vi "Status_Frame.vi"(8 "error in (no error)":errorcluster, 11 "Motor Control DevRef":T1={"DeviceStatus"={"status"=FALSE, "code"=0, "source"=""}, "Type"=enum."PWM", "PWM"={"PWM Channel"=enum."PWM 1", "DeadBand"={"Name"="", "maxPositivePwm"=0, "minPositivePwm"=0, "centerPwm"=0, "maxNegativePwm"=0, "minNegativePwm"=0, "angularRange"=0}}, "CAN"={"Device Number"=0, "SetOutput VI Ref"=variant(enum8{"Percent VBus", "Current", "Speed", "Position", "Voltage"} enum."Percent VBus"), "GetOutput VI Ref"=variant(refnum<k1> refnum), "Enable VI Ref"=variant(dbl 12.0), "Disable VI Ref"=variant(enum8{"Percent VBus", "Speed", "Position", "Slave", "Unchanged / Invalid", "Voltage Compensation", "Current", "Motion Profile"} enum."Percent VBus"), "Data"=variant}, "Invert"=FALSE, "DIO PWM"={"PWM \"Enable\" Channel"=enum."Invalid", "DIOChannel"=enum."Invalid", "PWM Rate"=0.0}}) -> (0 "error out":errorcluster, 3 "PhoenixMotorControlDevRef":T1={"DeviceStatus"={"status"=FALSE, "code"=0, "source"=""}, "Type"=enum."PWM", "PWM"={"PWM Channel"=enum."PWM 1", "DeadBand"={"Name"="", "maxPositivePwm"=0, "minPositivePwm"=0, "centerPwm"=0, "maxNegativePwm"=0, "minNegativePwm"=0, "angularRange"=0}}, "CAN"={"Device Number"=0, "SetOutput VI Ref"=variant(enum8{"Percent VBus", "Current", "Speed", "Position", "Voltage"} enum."Percent VBus"), "GetOutput VI Ref"=variant(refnum<k1> refnum), "Enable VI Ref"=variant(dbl 12.0), "Disable VI Ref"=variant(enum8{"Percent VBus", "Speed", "Position", "Slave", "Unchanged / Invalid", "Voltage Compensation", "Current", "Motion Profile"} enum."Percent VBus"), "Data"=variant}, "Invert"=FALSE, "DIO PWM"={"PWM \"Enable\" Channel"=enum."Invalid", "DIOChannel"=enum."Invalid", "PWM Rate"=0.0}})   [LabVIEW 2020]
uses:
  <vilib>/Rock Robotics/WPI/MotorControl/WPI_MotorControlDeviceRef.ctl
  <vilib>/Rock Robotics/WPI/MotorControl/WPI_MotorControlType.ctl
  <vilib>/Rock Robotics/SystemInterfaces/DIO/FPGA_DIOPWMChannel.ctl
  <vilib>/Rock Robotics/WPI/PWM/WPI_PWMDeadband.ctl
  <vilib>/Rock Robotics/SystemInterfaces/DIO/FPGA_DIOChannel.ctl
  <vilib>/Rock Robotics/WPI/ThirdParty/Phoenix-LabVIEW/Motor Controller/Controls/CTRE_Phoenix_MotorControl_StatusFrameEnhanced.ctl
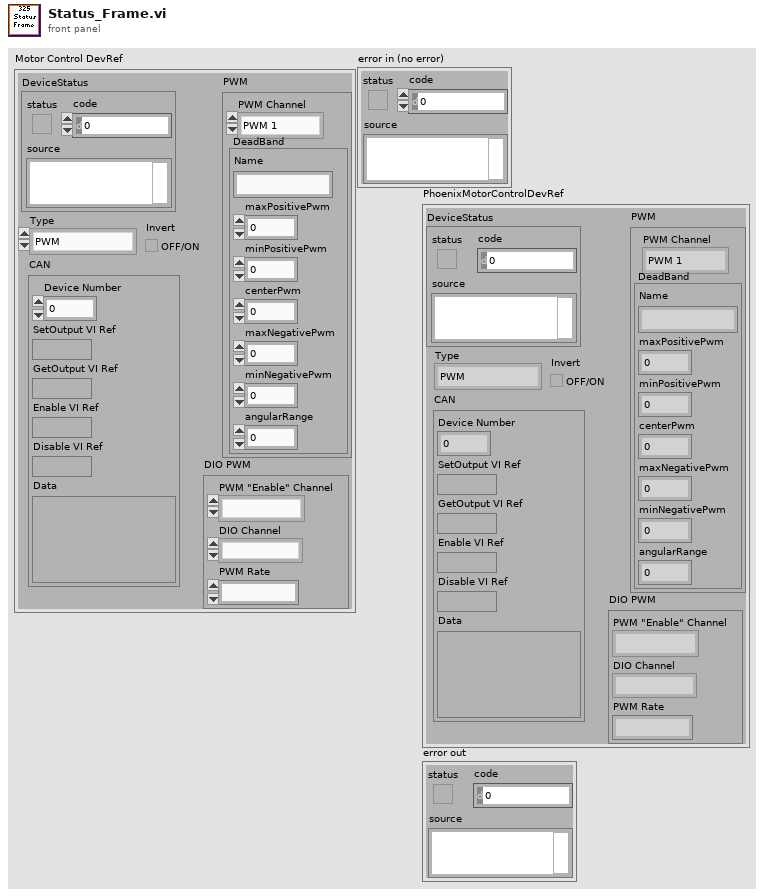
[diagram p1: front panel]
types:
  T1 = typedef "WPI_MotorControlDeviceRef.ctl" = cluster{"DeviceStatus":errorcluster, "Type":T2, "PWM":cluster{"PWM Channel":T3, "DeadBand":T4}, "CAN":cluster{"Device Number":u8, "SetOutput VI Ref":variant, "GetOutput VI Ref":variant, "Enable VI Ref":variant, "Disable VI Ref":variant, "Data":variant}, "Invert":bool, "DIO PWM":cluster{"PWM \"Enable\" Channel":T3, "DIOChannel":T5, "PWM Rate":dbl}}
  T2 = typedef "WPI_MotorControlType.ctl" = enum16{"PWM", "CAN", "DIO PWM"}
  T3 = typedef "FPGA_DIOPWMChannel.ctl" = enum8{"PWM 0", "PWM 1", "PWM 2", "PWM 3", "PWM 4", "PWM 5", "PWM 6", "PWM 7", "PWM 8", "PWM 9", "PWM MXP 0", "PWM MXP 1", "PWM MXP 2", "PWM MXP 3", "PWM MXP 4", "PWM MXP 5", "PWM MXP 6", "PWM MXP 7", "PWM MXP 8", "PWM MXP 9", "Invalid"}
  T4 = typedef "WPI_PWMDeadband.ctl" = cluster{"Name":string, "maxPositivePwm":i32, "minPositivePwm":i32, "centerPwm":i32, "maxNegativePwm":i32, "minNegativePwm":i32, "angularRange":u16}
  T5 = typedef "FPGA_DIOChannel.ctl" = enum8{"DIO 0", "DIO 1", "DIO 2", "DIO 3", "DIO 4", "DIO 5", "DIO 6", "DIO 7", "DIO 8", "DIO 9", "DIO MXP 0", "DIO MXP 1", "DIO MXP 2", "DIO MXP 3", "DIO MXP 4", "DIO MXP 5", "DIO MXP 6", "DIO MXP 7", "DIO MXP 8", "DIO MXP 9", "DIO MXP 10", "DIO MXP 11", "DIO MXP 12", "DIO MXP 13", "DIO MXP 14", "DIO MXP 15", "SPI Port CS1", "SPI Port CS2", "SPI Port CS3", "SPI Port MISO", "SPI Port MOSI", "Invalid"}
  T6 = typedef "CTRE_Phoenix_MotorControl_StatusFrameEnhanced.ctl" = u16
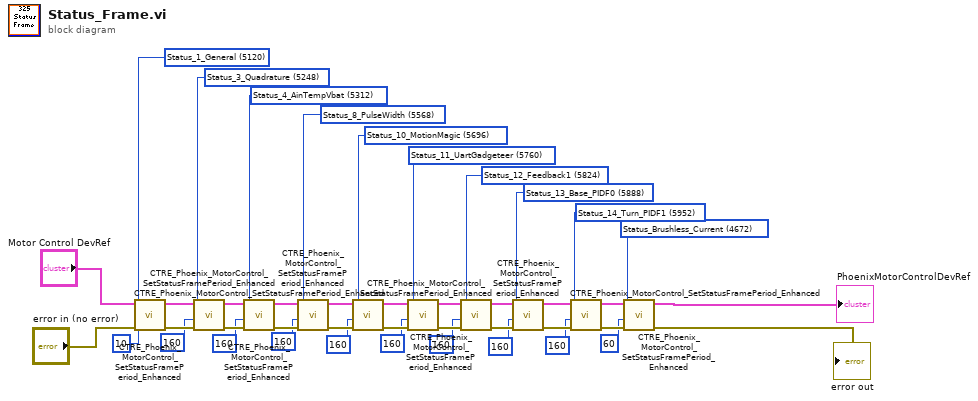
[diagram p0: block diagram]
diagram:
  w11 = T6 4672 items=["Status_1_General"=5120, "Status_2_Feedback0"=5184, "Status_3_Quadrature"=5248, "Status_4_AinTempVbat"=5312, "Status_6_Misc"=5440, "Status_7_CommStatus"=5504, "Status_8_PulseWidth"=5568, "Status_9_MotProfBuffer"=5632, "Status_10_MotionMagic"=5696, "Status_11_UartGadgeteer"=5760, "Status_12_Feedback1"=5824, "Status_13_Base_PIDF0"=5888, "Status_14_Turn_PIDF1"=5952, "Status_15_FirmwareApiStatus"=6016, "Status_Brushless_Current"=4672] ("Status Frame")
  w12 = T6 5952 items=["Status_1_General"=5120, "Status_2_Feedback0"=5184, "Status_3_Quadrature"=5248, "Status_4_AinTempVbat"=5312, "Status_6_Misc"=5440, "Status_7_CommStatus"=5504, "Status_8_PulseWidth"=5568, "Status_9_MotProfBuffer"=5632, "Status_10_MotionMagic"=5696, "Status_11_UartGadgeteer"=5760, "Status_12_Feedback1"=5824, "Status_13_Base_PIDF0"=5888, "Status_14_Turn_PIDF1"=5952, "Status_15_FirmwareApiStatus"=6016, "Status_Brushless_Current"=4672] ("Status Frame")
  w13 = T6 5888 items=["Status_1_General"=5120, "Status_2_Feedback0"=5184, "Status_3_Quadrature"=5248, "Status_4_AinTempVbat"=5312, "Status_6_Misc"=5440, "Status_7_CommStatus"=5504, "Status_8_PulseWidth"=5568, "Status_9_MotProfBuffer"=5632, "Status_10_MotionMagic"=5696, "Status_11_UartGadgeteer"=5760, "Status_12_Feedback1"=5824, "Status_13_Base_PIDF0"=5888, "Status_14_Turn_PIDF1"=5952, "Status_15_FirmwareApiStatus"=6016, "Status_Brushless_Current"=4672] ("Status Frame")
  w14 = T6 5824 items=["Status_1_General"=5120, "Status_2_Feedback0"=5184, "Status_3_Quadrature"=5248, "Status_4_AinTempVbat"=5312, "Status_6_Misc"=5440, "Status_7_CommStatus"=5504, "Status_8_PulseWidth"=5568, "Status_9_MotProfBuffer"=5632, "Status_10_MotionMagic"=5696, "Status_11_UartGadgeteer"=5760, "Status_12_Feedback1"=5824, "Status_13_Base_PIDF0"=5888, "Status_14_Turn_PIDF1"=5952, "Status_15_FirmwareApiStatus"=6016, "Status_Brushless_Current"=4672] ("Status Frame")
  w15 = T6 5760 items=["Status_1_General"=5120, "Status_2_Feedback0"=5184, "Status_3_Quadrature"=5248, "Status_4_AinTempVbat"=5312, "Status_6_Misc"=5440, "Status_7_CommStatus"=5504, "Status_8_PulseWidth"=5568, "Status_9_MotProfBuffer"=5632, "Status_10_MotionMagic"=5696, "Status_11_UartGadgeteer"=5760, "Status_12_Feedback1"=5824, "Status_13_Base_PIDF0"=5888, "Status_14_Turn_PIDF1"=5952, "Status_15_FirmwareApiStatus"=6016, "Status_Brushless_Current"=4672] ("Status Frame")
  w16 = T6 5696 items=["Status_1_General"=5120, "Status_2_Feedback0"=5184, "Status_3_Quadrature"=5248, "Status_4_AinTempVbat"=5312, "Status_6_Misc"=5440, "Status_7_CommStatus"=5504, "Status_8_PulseWidth"=5568, "Status_9_MotProfBuffer"=5632, "Status_10_MotionMagic"=5696, "Status_11_UartGadgeteer"=5760, "Status_12_Feedback1"=5824, "Status_13_Base_PIDF0"=5888, "Status_14_Turn_PIDF1"=5952, "Status_15_FirmwareApiStatus"=6016, "Status_Brushless_Current"=4672] ("Status Frame")
  w17 = T6 5568 items=["Status_1_General"=5120, "Status_2_Feedback0"=5184, "Status_3_Quadrature"=5248, "Status_4_AinTempVbat"=5312, "Status_6_Misc"=5440, "Status_7_CommStatus"=5504, "Status_8_PulseWidth"=5568, "Status_9_MotProfBuffer"=5632, "Status_10_MotionMagic"=5696, "Status_11_UartGadgeteer"=5760, "Status_12_Feedback1"=5824, "Status_13_Base_PIDF0"=5888, "Status_14_Turn_PIDF1"=5952, "Status_15_FirmwareApiStatus"=6016, "Status_Brushless_Current"=4672] ("Status Frame")
  w18 = T6 5312 items=["Status_1_General"=5120, "Status_2_Feedback0"=5184, "Status_3_Quadrature"=5248, "Status_4_AinTempVbat"=5312, "Status_6_Misc"=5440, "Status_7_CommStatus"=5504, "Status_8_PulseWidth"=5568, "Status_9_MotProfBuffer"=5632, "Status_10_MotionMagic"=5696, "Status_11_UartGadgeteer"=5760, "Status_12_Feedback1"=5824, "Status_13_Base_PIDF0"=5888, "Status_14_Turn_PIDF1"=5952, "Status_15_FirmwareApiStatus"=6016, "Status_Brushless_Current"=4672] ("Status Frame")
  w19 = T6 5248 items=["Status_1_General"=5120, "Status_2_Feedback0"=5184, "Status_3_Quadrature"=5248, "Status_4_AinTempVbat"=5312, "Status_6_Misc"=5440, "Status_7_CommStatus"=5504, "Status_8_PulseWidth"=5568, "Status_9_MotProfBuffer"=5632, "Status_10_MotionMagic"=5696, "Status_11_UartGadgeteer"=5760, "Status_12_Feedback1"=5824, "Status_13_Base_PIDF0"=5888, "Status_14_Turn_PIDF1"=5952, "Status_15_FirmwareApiStatus"=6016, "Status_Brushless_Current"=4672] ("Status Frame")
  w20 = T6 5120 items=["Status_1_General"=5120, "Status_2_Feedback0"=5184, "Status_3_Quadrature"=5248, "Status_4_AinTempVbat"=5312, "Status_6_Misc"=5440, "Status_7_CommStatus"=5504, "Status_8_PulseWidth"=5568, "Status_9_MotProfBuffer"=5632, "Status_10_MotionMagic"=5696, "Status_11_UartGadgeteer"=5760, "Status_12_Feedback1"=5824, "Status_13_Base_PIDF0"=5888, "Status_14_Turn_PIDF1"=5952, "Status_15_FirmwareApiStatus"=6016, "Status_Brushless_Current"=4672] ("Status Frame")
  n1 = call <vilib>:"CTRE_Phoenix_MotorControl_SetStatusFramePeriod_Enhanced.vi"("error in (no error)"="error in (no error)", "periodMs"=10, "Status Frame"=w20, "PhoenixMotorControlDevRef"="Motor Control DevRef") -> ("error out"=w34:errorcluster, "PhoenixMotorControlDevRef"=w33:T1)  [unwired: 6 in]
  n2 = call <vilib>:"CTRE_Phoenix_MotorControl_SetStatusFramePeriod_Enhanced.vi"("error in (no error)"=w34, "periodMs"=160, "Status Frame"=w19, "PhoenixMotorControlDevRef"=w33) -> ("error out"=w35:errorcluster, "PhoenixMotorControlDevRef"=w32:T1)  [unwired: 6 in]
  n3 = call <vilib>:"CTRE_Phoenix_MotorControl_SetStatusFramePeriod_Enhanced.vi"("error in (no error)"=w35, "periodMs"=160, "Status Frame"=w18, "PhoenixMotorControlDevRef"=w32) -> ("error out"=w36:errorcluster, "PhoenixMotorControlDevRef"=w31:T1)  [unwired: 6 in]
  n4 = call <vilib>:"CTRE_Phoenix_MotorControl_SetStatusFramePeriod_Enhanced.vi"("error in (no error)"=w36, "periodMs"=160, "Status Frame"=w17, "PhoenixMotorControlDevRef"=w31) -> ("error out"=w37:errorcluster, "PhoenixMotorControlDevRef"=w30:T1)  [unwired: 6 in]
  n5 = call <vilib>:"CTRE_Phoenix_MotorControl_SetStatusFramePeriod_Enhanced.vi"("error in (no error)"=w37, "periodMs"=160, "Status Frame"=w16, "PhoenixMotorControlDevRef"=w30) -> ("error out"=w42:errorcluster, "PhoenixMotorControlDevRef"=w29:T1)  [unwired: 6 in]
  n6 = call <vilib>:"CTRE_Phoenix_MotorControl_SetStatusFramePeriod_Enhanced.vi"("error in (no error)"=w42, "periodMs"=160, "Status Frame"=w15, "PhoenixMotorControlDevRef"=w29) -> ("error out"=w38:errorcluster, "PhoenixMotorControlDevRef"=w28:T1)  [unwired: 6 in]
  n7 = call <vilib>:"CTRE_Phoenix_MotorControl_SetStatusFramePeriod_Enhanced.vi"("error in (no error)"=w38, "periodMs"=160, "Status Frame"=w14, "PhoenixMotorControlDevRef"=w28) -> ("error out"=w39:errorcluster, "PhoenixMotorControlDevRef"=w27:T1)  [unwired: 6 in]
  n8 = call <vilib>:"CTRE_Phoenix_MotorControl_SetStatusFramePeriod_Enhanced.vi"("error in (no error)"=w39, "periodMs"=160, "Status Frame"=w13, "PhoenixMotorControlDevRef"=w27) -> ("error out"=w40:errorcluster, "PhoenixMotorControlDevRef"=w26:T1)  [unwired: 6 in]
  n9 = call <vilib>:"CTRE_Phoenix_MotorControl_SetStatusFramePeriod_Enhanced.vi"("error in (no error)"=w40, "periodMs"=160, "Status Frame"=w12, "PhoenixMotorControlDevRef"=w26) -> ("error out"=w41:errorcluster, "PhoenixMotorControlDevRef"=w25:T1)  [unwired: 6 in]
  n10 = call <vilib>:"CTRE_Phoenix_MotorControl_SetStatusFramePeriod_Enhanced.vi"("error in (no error)"=w41, "periodMs"=60, "Status Frame"=w11, "PhoenixMotorControlDevRef"=w25) -> ("error out"=→"error out":errorcluster, "PhoenixMotorControlDevRef"=→"PhoenixMotorControlDevRef":T1)  [unwired: 6 in]
